vi "Measure Output Voltage.vi"(7 "Slave Address":i32=-1 min=-1 max=30 step=1, 8 "error":errorcluster, 11 "VISA":refnum<visa-resource-name>) -> (0 "error out":errorcluster, 2 "Output Voltage":dbl format="%.4f", 3 "VISA out":refnum<visa-resource-name>)   [LabVIEW 2025, in "TDK-Lambda GEN LAN Series.lvlib"]
doc: "Reads the output voltage as measured by the power supply."
uses:
  <userlib>/TDK-Lambda GEN LAN Series/TDK-Lambda GEN LAN Series.lvlib
panel:
  # "TDK-Lambda Genesys \n LAN\n  DC Power Supplies"
  # "Measure the \nOutput Voltage"
  # "(c) 2019 TDK-Lambda.  ALL RIGHTS RESERVED."
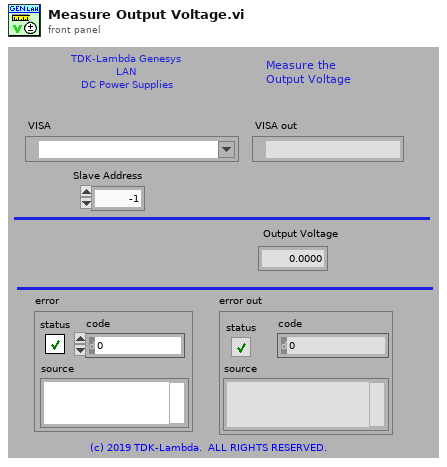
[diagram p1: front panel]
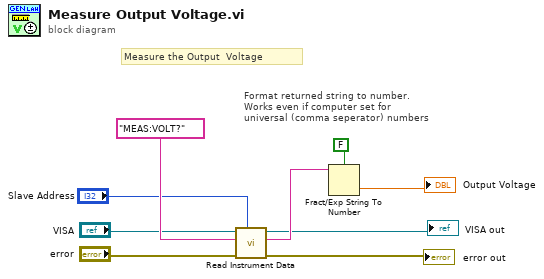
[diagram p0: block diagram]
diagram:
  # "Format returned string to number.\nWorks even if computer set for \nuniversal (comma seperator) numbers"
  # "Measure the Output  Voltage"
  n1 = call <userlib>:"Read Instrument Data.vi"("Slave Address"="Slave Address", "error"="error", "Query"="MEAS:VOLT?" ("format string"), "VISA"="VISA") -> ("error out"=→"error out":errorcluster, "Response"=w7:string, "VISA out"=→"VISA out":refnum<visa-resource-name>)  [unwired: 4 in, 1 out]
  n2 = Fract/Exp String To Number(use system decimal point (T)=FALSE, string=w7) -> (number=→"Output Voltage":dbl)  [unwired: 2 in, 1 out]
